vi "告警码字段定义.vi"(10 "首次调用？":bool, 11 "告警代码":u16(ring) items=["无告警", "缺试剂告警", "缺水样告警", "缺蒸馏水告警", "缺标液告警", "仪表漏液告警", "标定异常告警", "超量程告警", "加热异常", "低试剂预警", "超上限告警", "超下限告警", "仪表内部其他异常"]) -> (3 "data":T1)   [LabVIEW 2016, in "挥发酚.lvlib"]
uses:
  Alarm interface/Alarm interface.lvlib
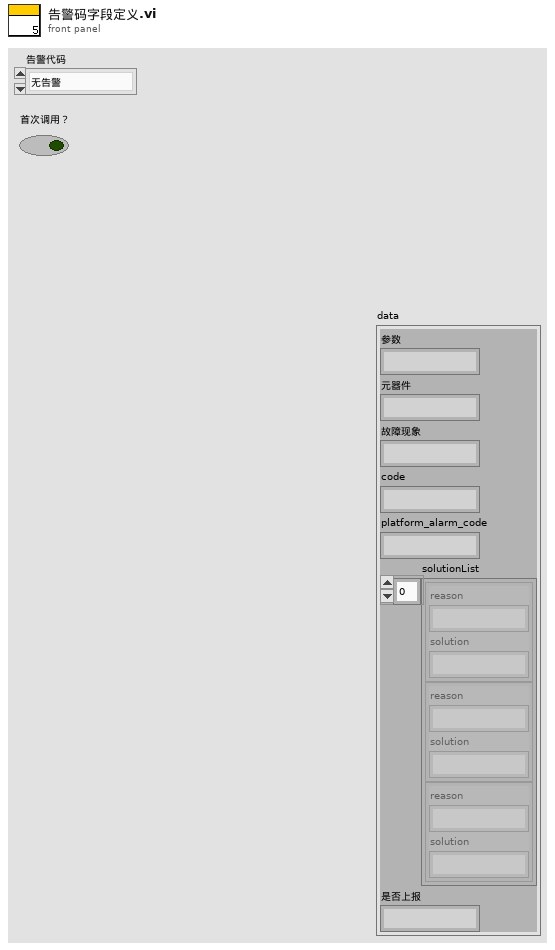
[diagram p1: front panel]
types:
  T1 = typedef "Alarm interface.lvlib/报警短信语音交互.ctl" = cluster{"参数":string, "元器件":string, "故障现象":string, "code":string, "platform_alarm_code":string, "solutionList":cluster{"reason":string, "solution":string}[], "是否上报":string}
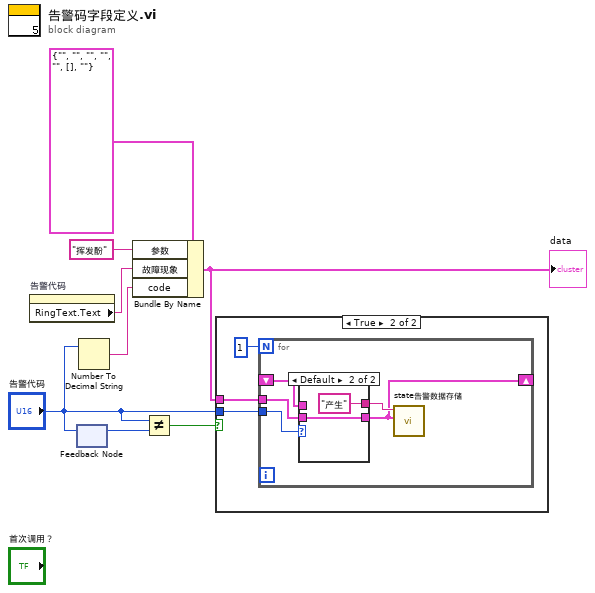
[diagram p0: block diagram]
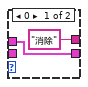
[diagram p3: hidden frame]
diagram:
  n1 = property on="告警代码" class="Ring (strict)"() -> ("RingText.Text"=w6:string)  [unwired: 2 in, 2 out]
  n2 = feedback #1() -> (w4:u16)  [unwired: 1 in]
  n3 = feedback-in #1("告警代码") -> ()
  n4 = Number To Decimal String(number="告警代码") -> (decimal integer string=w5:string)  [unwired: 1 in]
  n5 = Bundle By Name(cluster=T1 {"参数"="", "元器件"="", "故障现象"="", "code"="", "platform_alarm_code"="", "solutionList"=[], "是否上报"=""} ("data"), "参数"="挥发酚", "故障现象"=w6, "code"=w5) -> (w1:T1)
  "data" <- w1
  n6 = Not Equal?(x="告警代码", y=w4) -> (x != y?=w3:bool)
  n7 = case shown="True" w3 {
    tunnel: "告警代码" -> [_ w11]
    tunnel: w1 -> [_ w10]
    frame False {
    }
    frame True {
      n8 = for {
        N: 1 -> [_]
        tunnel: w11 -> [w16]
        shift-right: [w12] -> _
        shift-left: _ -> [w14]
        tunnel: w10 -> [w13]
        n9 = case shown="Default" w16 {
          tunnel: ["消除" "产生"] -> w15
          tunnel: w14 -> [w17 _]
          tunnel: [w17 w19] -> w12
          tunnel: w13 -> [_ w19]
          frame 0 {
          }
          frame Default {
          }
        }
        n10 = call "state告警数据存储.vi"("data"=w12, "state"=w15) -> ()  [unwired: 9 in, 1 out]
      }
    }
  }
